vi "RunTillAbort - Luca.vi"(0 "Exposure Time (secs)":sgl, 1 "EM Advanced":i32 min=0 max=300 step=1, 2 "EM Gain":i32=1 min=1 max=300 step=1, 3 "Readout Speed (MHz)":i32 min=0 max=0, 5 "Trigger Mode":T1, 6 "Start Acquisition":bool, 8 "stop":bool, 10 "shutdown":bool) -> (4 "VS Speed (us)":sgl format="%.2f", 7 "Start Acquisition":bool, 9 "Acquiring":bool, 11 "Shut Down":bool, 19 "Intensity Graph":i32[][](graph))   [LabVIEW 2013]
uses:
  System Files/user.lib/atmcd32d.llb/TriggerMode_mode typedef.ctl
  System Files/user.lib/atmcd32d.llb/HSSpeed_type typedef.ctl
  System Files/user.lib/atmcd32d.llb/EMGainMode_mode typedef.ctl
  System Files/user.lib/atmcd32d.llb/Error Code Enum typedef.ctl
  System Files/user.lib/atmcd32d.llb/Shutter_type typedef.ctl
  System Files/user.lib/atmcd32d.llb/Shutter_mode typedef.ctl
panel:
  out "Cycle Time":sgl format="%.4f"
  out "Temperature Stable":bool
  out "Current Temperature":i32
  in  "VS Speed (us)":i32 min=0 max=0
  out "Readout Speed (MHz)":sgl format="%.2f"
  out "Start Acquisition":u32
  out "SetTriggerMode":u32
  out "SetVSSpeed":u32
  out "SetHSSpeed":u32
  out "GetMostRecentImage":u32
  out "Image Array":i32[](array[numeric]) caption="Array"
  out "Shutdown":u32
  out "GetDetector":u32
  out "Y Pixels":i32
  out "Total number of pixels":i32
  out "SetImage":u32
  out "X Pixels":i32
  out "SetExposureTime":u32
  out "SetReadMode":u32
  out "SetAcquisition Mode":u32
  out "Initialize":u32
  # "Return Values"
  # "Numerical data"
  # "INPUT"
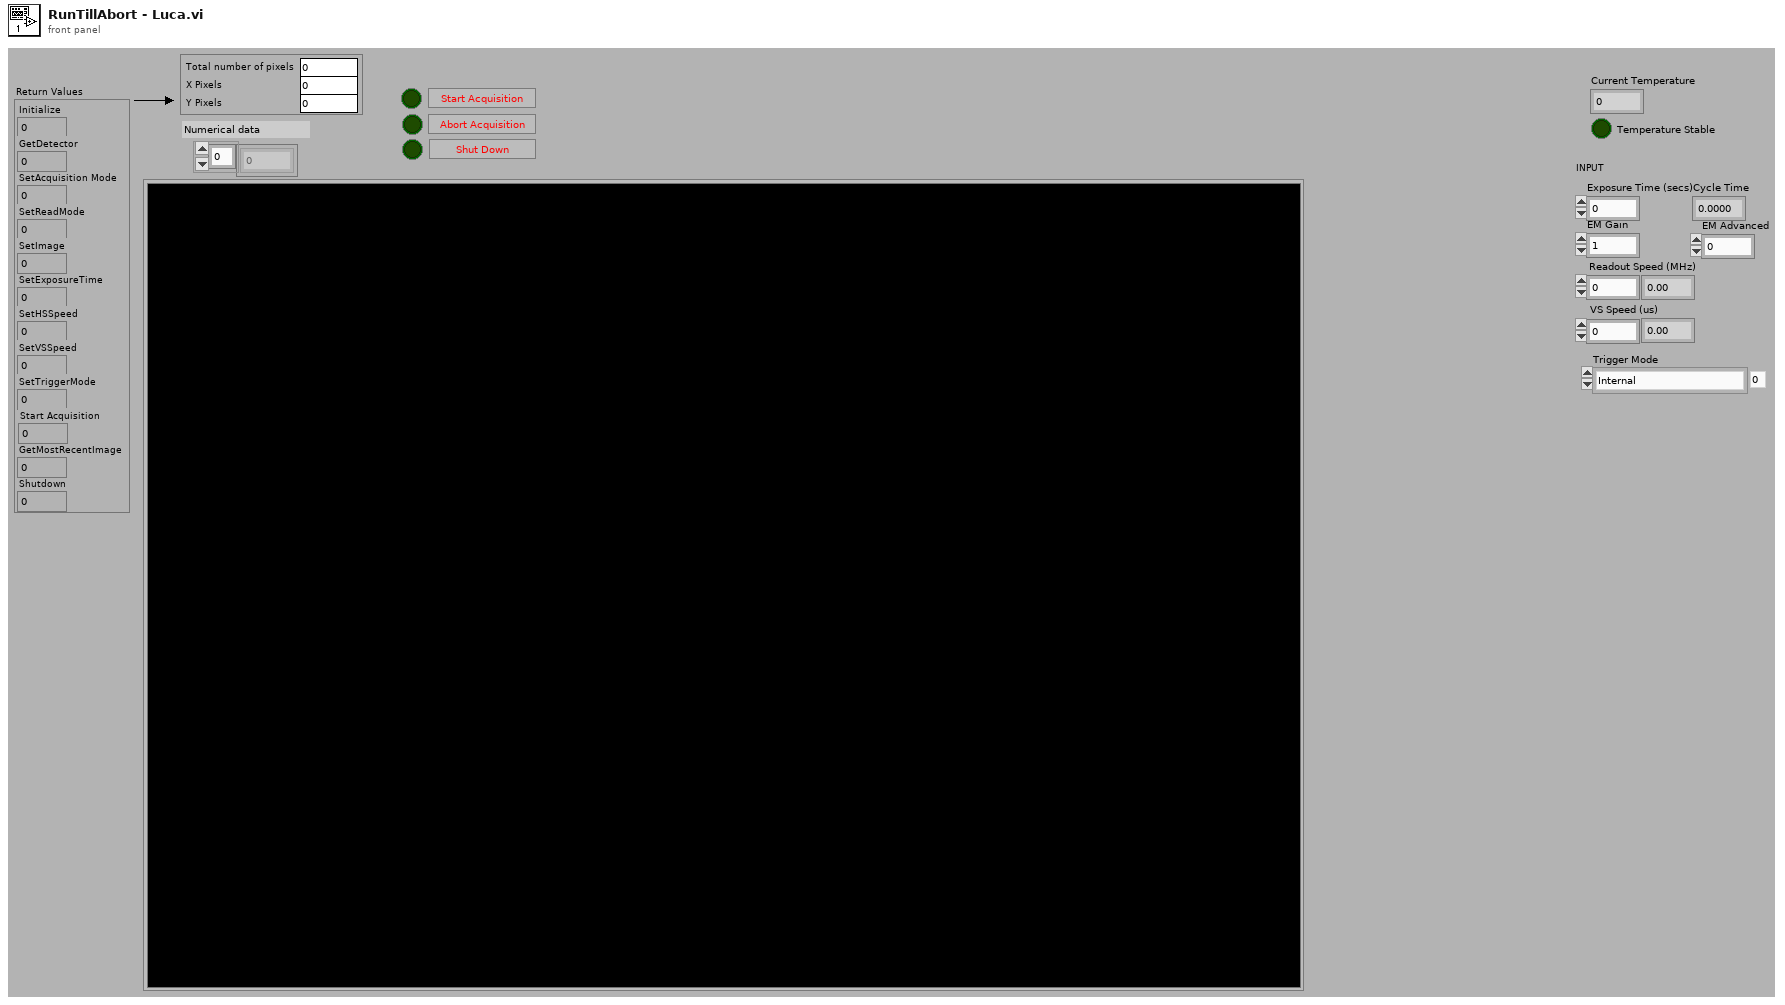
[diagram p1: front panel]
types:
  T1 = typedef "TriggerMode_mode typedef.ctl" = enum16{"Internal", "External", "N/A (2)", "N/A (3)", "N/A (4)", "N/A (5)", "External Start", "External Exposure (Bulb)", "N/A (8)", "External FVB EM", "Software", "N/A (11)", "External Charge Shifting"}
  T2 = typedef "EMGainMode_mode typedef.ctl" = enum16{"8-bit", "12-bit", "Linear", "Real"}
  T3 = typedef "Error Code Enum typedef.ctl" = enum32{"N/A (0)", "DRV_ERROR_CODES", "DRV_SUCCESS", "DRV_VXDNOTINSTALLED", "DRV_ERROR_SCAN", "DRV_ERROR_CHECK_SUM", "DRV_ERROR_FILELOAD", "DRV_UNKNOWN_FUNC", "DRV_ERROR_VXD_INIT", "DRV_ERROR_ADDRESS", "DRV_ERROR_PAGELOCK", "DRV_ERROR_PAGEUNLOCK", "DRV_ERROR_BOARDTEST", "DRV_ERROR_ACK", "DRV_ERROR_UP_FIFO", "DRV_ERROR_PATTERN", "N/A (16)", "DRV_ACQUISITION_ERRORS", "DRV_ACQ_BUFFER", "DRV_ACQ_DOWNFIFO_FULL", "DRV_PROC_UNKONWN_INSTRUCTION", "DRV_ILLEGAL_OP_CODE", "DRV_KINETIC_TIME_NOT_MET", "DRV_ACCUM_TIME_NOT_MET", "DRV_NO_NEW_DATA", "N/A (25)", "DRV_SPOOLERROR", "N/A (27)", "N/A (28)", "N/A (29)", "N/A (30)", "N/A (31)", "N/A (32)", "DRV_TEMPERATURE_CODES", "DRV_TEMPERATURE_OFF", "DRV_TEMPERATURE_NOT_STABILIZED", "DRV_TEMPERATURE_STABILIZED", "DRV_TEMPERATURE_NOT_REACHED", "DRV_TEMPERATURE_OUT_RANGE", "DRV_TEMPERATURE_NOT_SUPPORTED", "DRV_TEMPERATURE_DRIFT", "N/A (41)", "N/A (42)", "N/A (43)", "N/A (44)", "N/A (45)", "N/A (46)", "N/A (47)", "N/A (48)", "DRV_GENERAL_ERRORS", "DRV_INVALID_AUX", "DRV_COF_NOTLOADED", "DRV_FPGAPROG", "DRV_FLEXERROR", "DRV_GPIBERROR", "N/A (55)", "N/A (56)", "N/A (57)", "N/A (58)", "N/A (59)", "N/A (60)", "N/A (61)", "N/A (62)", "N/A (63)", "DRV_DATATYPE", "DRV_DRIVER_ERRORS", "DRV_P1INVALID", "DRV_P2INVALID", "DRV_P3INVALID", "DRV_P4INVALID", "DRV_INIERROR", "DRV_COFERROR", "DRV_ACQUIRING", "DRV_IDLE", "DRV_TEMPCYCLE", "DRV_NOT_INITIALIZED", "DRV_P5INVALID", "DRV_P6INVALID", "DRV_INVALID_MODE", "DRV_INVALID_FILTER", "DRV_I2CERRORS", "DRV_I2CDEVNOTFOUND", "DRV_I2CTIMEOUT", "DRV_P7INVALID", "N/A (84)", "N/A (85)", "N/A (86)", "N/A (87)", "N/A (88)", "N/A (89)", "DRV_IOCERROR", "DRV_VRMVERSIONERROR"}
  T4 = typedef "Shutter_mode typedef.ctl" = enum16{"Auto", "Open", "Close"}
  T5 = typedef "Shutter_type typedef.ctl" = enum16{"TTL Low", "TTL High"}
  T6 = typedef "HSSpeed_type typedef.ctl" = enum16{"EM Amp", "Conventional Amp"}
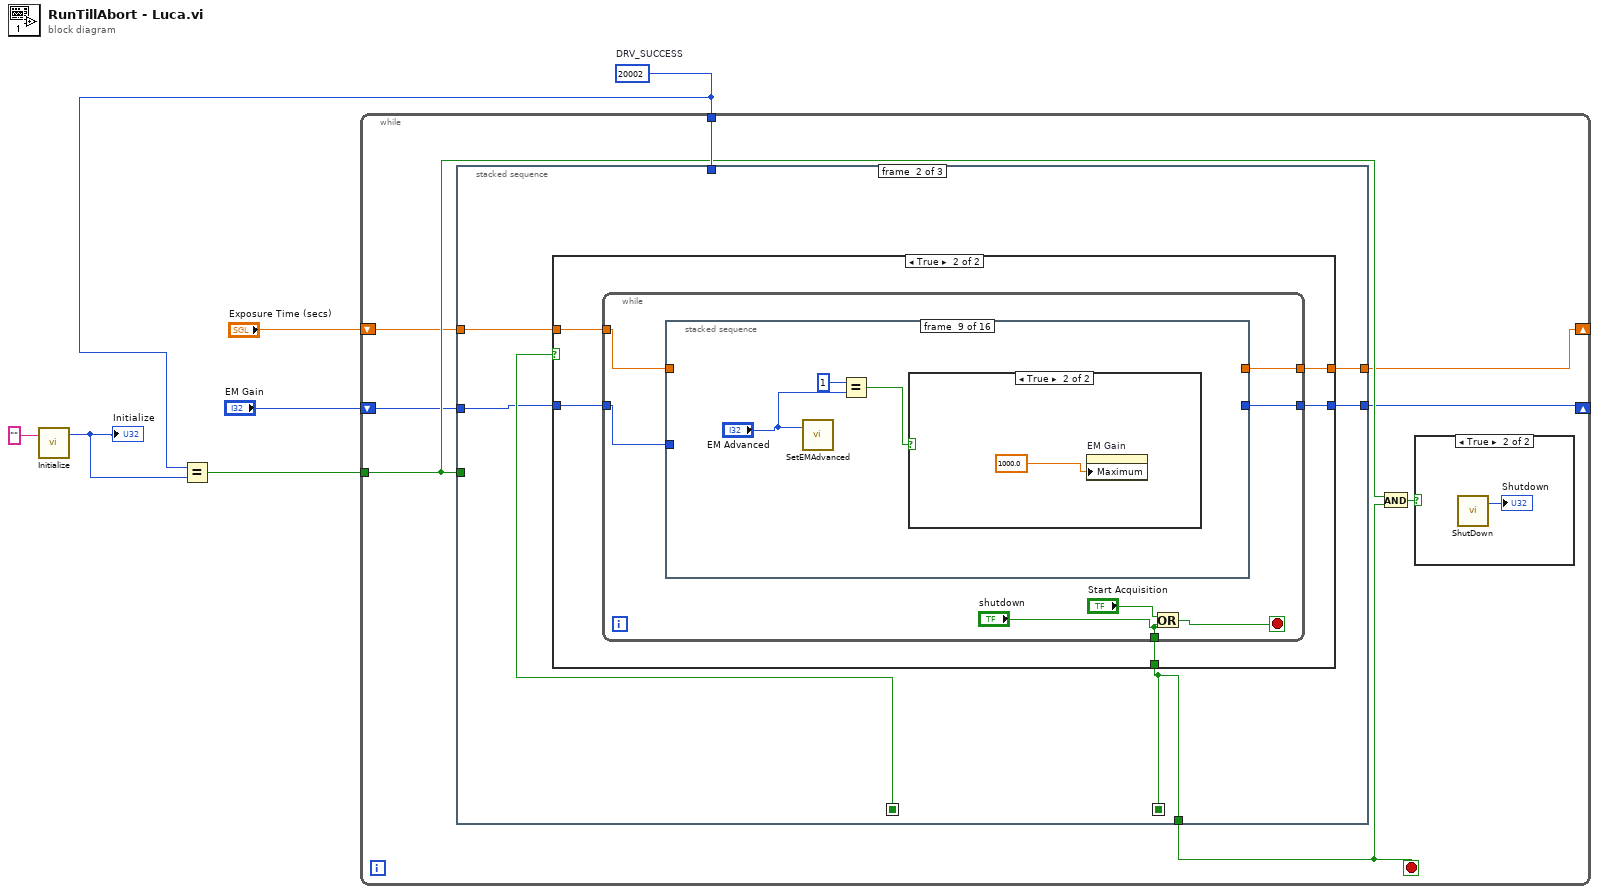
[diagram p0: block diagram]
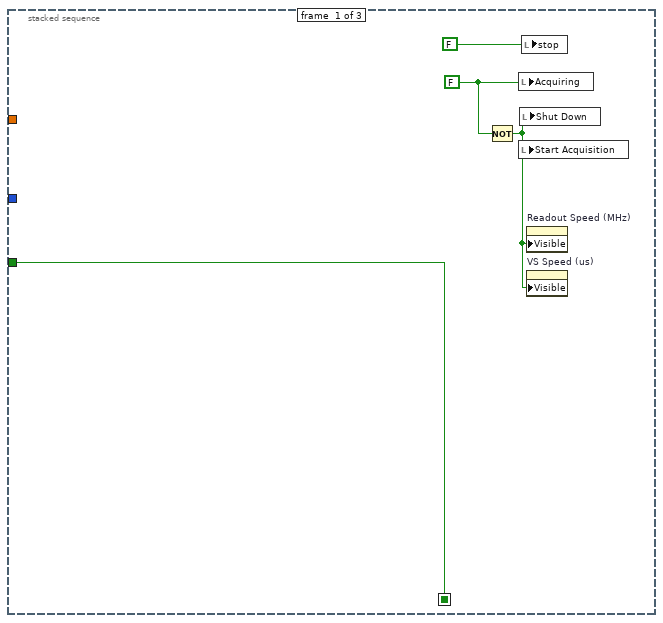
[diagram p3: hidden frame]
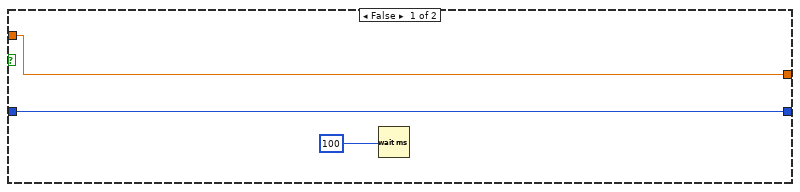
[diagram p4: hidden frame]
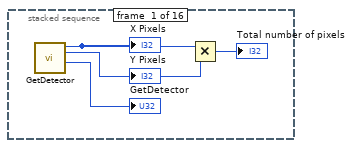
[diagram p5: hidden frame]
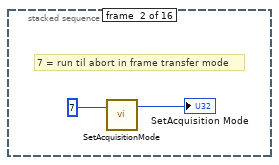
[diagram p6: hidden frame]
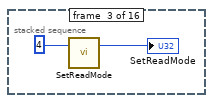
[diagram p7: hidden frame]
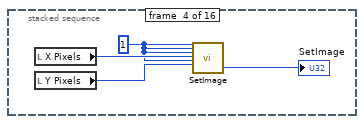
[diagram p8: hidden frame]
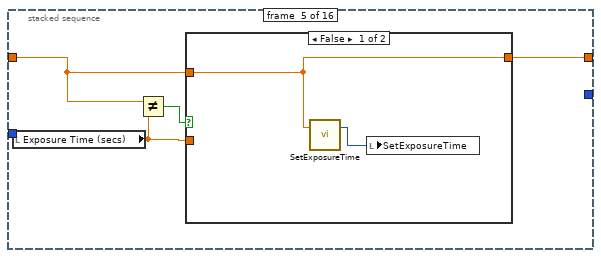
[diagram p9: hidden frame]
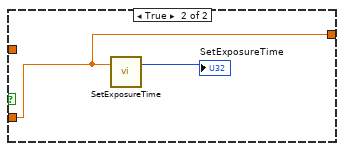
[diagram p10: hidden frame]
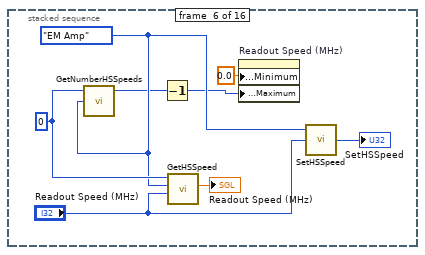
[diagram p11: hidden frame]
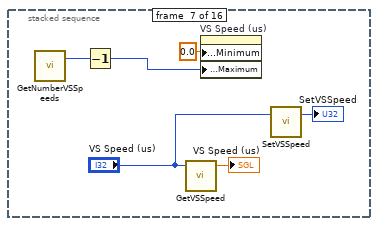
[diagram p12: hidden frame]
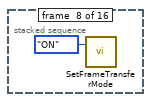
[diagram p13: hidden frame]
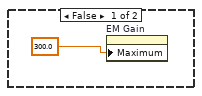
[diagram p14: hidden frame]
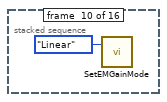
[diagram p15: hidden frame]
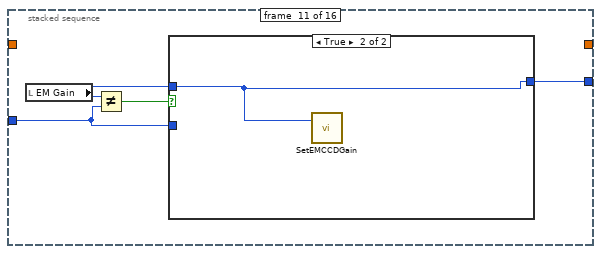
[diagram p16: hidden frame]
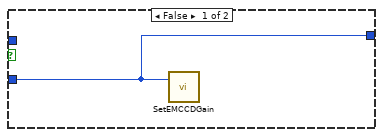
[diagram p17: hidden frame]
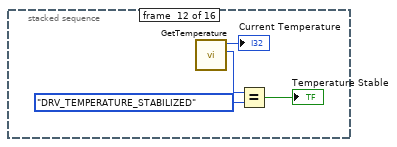
[diagram p18: hidden frame]
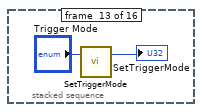
[diagram p19: hidden frame]
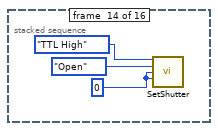
[diagram p20: hidden frame]
diagram:
  w3 = 20002  # DRV_SUCCESS
  n1 = call "Initialize.vi"("directory (\"\")"="") -> ("DLL error code"=w6:u32)  [unwired: 1 in, 1 out]
  "Initialize" <- w6
  n2 = Equal?(x=w3, y=w6) -> (x = y?=w4:bool)
  n3 = while {
    tunnel: w3 -> [w14]
    tunnel: w4 -> [w11]
    shift-right: [w8] -> _
    shift-left: "Exposure Time (secs)" -> [w10]
    shift-right: [w7] -> _
    shift-left: "EM Gain" -> [w9]
    stop <- w12 stop-if-true
    n4 = stacked-sequence {
      seq-local: [w18 _ _] -> [_ w25 w102]
      seq-local: [_ w22 _] -> [_ _ w104]
      tunnel: w14 -> [_ _ w107]
      tunnel: w9 -> [_ w24 w106]
      tunnel: w10 -> [_ w23 w105]
      tunnel: [_ w22 _] -> w12
      tunnel: w11 -> [w18 _ _]
      tunnel: [_ w21 _] -> w8
      tunnel: [_ w20 _] -> w7
      frame #0 {
        w17 = FALSE
        n5 = Not(x=w17) -> (.not. x?=w16:bool)
        n6 = local write "Acquiring"(w17) -> ()
        n7 = local write "Start Acquisition"(w16) -> ()
        n8 = local write "Shut Down"(w16) -> ()
        n9 = local write "stop"(FALSE) -> ()
        n10 = property on="Readout Speed (MHz)" class="DigNum (strict)"("Visible"=w16) -> ()  [unwired: 2 in, 2 out]
        n11 = property on="VS Speed (us)" class="DigNum (strict)"("Visible"=w16) -> ()  [unwired: 2 in, 2 out]
      }
      frame #1 {
        n12 = case shown="True" w25 {
          tunnel: w24 -> [w26 w33]
          tunnel: w23 -> [w27 w32]
          tunnel: [_ w31] -> w22
          tunnel: [w27 w30] -> w21
          tunnel: [w26 w29] -> w20
          frame False {
            n13 = Wait (ms)(milliseconds to wait=100) -> ()  [unwired: 1 out]
          }
          frame True {
            n14 = while {
              tunnel: w33 -> [w40]
              tunnel: w32 -> [w39]
              tunnel: ["shutdown"] -> w31
              tunnel: [w35] -> w30
              tunnel: [w34] -> w29
              stop <- w37 stop-if-true
              n15 = stacked-sequence {
                tunnel: w40 -> [_ _ _ _ _ _ _ _ _ _ w83 _ _ _ _ _]
                tunnel: w39 -> [_ _ _ _ w53 _ _ _ _ _ _ _ _ _ _ _]
                tunnel: [_ _ _ _ w54 _ _ _ _ _ _ _ _ _ _ _] -> w35
                tunnel: [_ _ _ _ _ _ _ _ _ _ w82 _ _ _ _ _] -> w34
                frame #0 {
                  n16 = call "GetDetector.vi"() -> ("DLL error code"=→"GetDetector":u32, "ypixels"=w43:i32, "xpixels"=w42:i32)  [unwired: 4 in, 1 out]
                  "X Pixels" <- w42
                  "Y Pixels" <- w43
                  n17 = Multiply(x=w42, y=w43) -> (x*y=→"Total number of pixels":i32)
                }
                frame #1 {
                  # "7 = run til abort in frame transfer mode"
                  n18 = call "SetAcquisitionMode.vi"("mode"=u16 7 ("AcquisitionMode")) -> ("DLL error code"=→"SetAcquisition Mode":u32)  [unwired: 1 in, 1 out]
                }
                frame #2 {
                  n19 = call "SetReadMode.vi"("mode"=u16 4 ("ReadMode")) -> ("DLL error code"=→"SetReadMode":u32)  [unwired: 1 in, 1 out]
                }
                frame #3 {
                  w51 = 1
                  n20 = local read "X Pixels"() -> (w52:i32)
                  n21 = local read "Y Pixels"() -> (w50:i32)
                  n22 = call "SetImage.vi"("hbin"=w51, "vbin"=w51, "hstart"=w51, "hend"=w52, "vstart"=w51, "vend"=w50) -> ("DLL error code"=→"SetImage":u32)  [unwired: 20 in, 1 out]
                }
                frame #4 {
                  n23 = local read "Exposure Time (secs)"() -> (w55:sgl)
                  n24 = Not Equal?(x=w53, y=w55) -> (x != y?=w56:bool)
                  n25 = case shown="False" w56 {
                    tunnel: w55 -> [_ w59]
                    tunnel: [w57 w59] -> w54
                    tunnel: w53 -> [w57 _]
                    frame False {
                      n26 = call "SetExposureTime.vi"("time"=w57) -> ("DLL error code"=w58:u32)  [unwired: 1 in, 1 out]
                      n27 = local write "SetExposureTime"(w58) -> ()
                    }
                    frame True {
                      n28 = call "SetExposureTime.vi"("time"=w59) -> ("DLL error code"=→"SetExposureTime":u32)  [unwired: 1 in, 1 out]
                    }
                  }
                }
                frame #5 {
                  w67 = 0 ("channel")
                  w66 = HSSpeed_type_typedef."EM Amp" ("type")
                  n29 = call "GetNumberHSSpeeds.vi"("type"=w66, "channel"=w67) -> ("number"=w64:i32)  [unwired: 1 in, 2 out]
                  n30 = Decrement(x=w64) -> (x-1=w63:i32)
                  n31 = call "GetHSSpeed.vi"("index"="Readout Speed (MHz)", "type"=w66, "channel"=w67) -> ("speed"=→"Readout Speed (MHz)":sgl)  [unwired: 2 in, 2 out]
                  n32 = property on="Readout Speed (MHz)" class="DigNum (strict)"("Data Range:Minimum"=0.0, "Data Range:Maximum"=w63) -> ()  [unwired: 2 in, 2 out]
                  n33 = call "SetHSSpeed.vi"("index"="Readout Speed (MHz)", "type"=w66) -> ("DLL error code"=→"SetHSSpeed":u32)  [unwired: 2 in, 1 out]
                }
                frame #6 {
                  n34 = call "GetNumberVSSpeeds.vi"() -> ("number"=w69:i32)  [unwired: 3 in, 2 out]
                  n35 = Decrement(x=w69) -> (x-1=w70:i32)
                  n36 = call "GetVSSpeed.vi"("index"="VS Speed (us)") -> ("speed"=→"VS Speed (us)":sgl)  [unwired: 2 in, 2 out]
                  n37 = property on="VS Speed (us)" class="DigNum (strict)"("Data Range:Minimum"=0.0, "Data Range:Maximum"=w70) -> ()  [unwired: 2 in, 2 out]
                  n38 = call "SetVSSpeed.vi"("index"="VS Speed (us)") -> ("DLL error code"=→"SetVSSpeed":u32)  [unwired: 1 in, 1 out]
                }
                frame #7 {
                  n39 = call "SetFrameTransferMode.vi"("mode"=enum16{"OFF", "ON"}."ON") -> ()  [unwired: 1 in, 2 out]
                }
                frame #8 {
                  n40 = call "SetEMAdvanced.vi"("state"="EM Advanced") -> ()  [unwired: 1 in, 2 out]
                  n41 = Equal?(x=1, y="EM Advanced") -> (x = y?=w78:bool)
                  n42 = case shown="True" w78 {
                    frame False {
                      n43 = property on="EM Gain" class="DigNum (strict)"("Maximum"=300.0 ("Data Range:Maximum")) -> ()  [unwired: 2 in, 2 out]
                    }
                    frame True {
                      n44 = property on="EM Gain" class="DigNum (strict)"("Maximum"=1000.0 ("Data Range:Maximum")) -> ()  [unwired: 2 in, 2 out]
                    }
                  }
                }
                frame #9 {
                  n45 = call "SetEMGainMode.vi"("mode"=EMGainMode_mode_typedef."Linear") -> ()  [unwired: 1 in, 2 out]
                }
                frame #10 {
                  n46 = local read "EM Gain"() -> (w84:i32)
                  n47 = Not Equal?(x=w84, y=w83) -> (x != y?=w85:bool)
                  n48 = case shown="True" w85 {
                    tunnel: w84 -> [_ w87]
                    tunnel: w83 -> [w86 _]
                    tunnel: [w86 w87] -> w82
                    frame False {
                      n49 = call "SetEMCCDGain.vi"("gain"=w86) -> ()  [unwired: 1 in, 2 out]
                    }
                    frame True {
                      n50 = call "SetEMCCDGain.vi"("gain"=w87) -> ()  [unwired: 1 in, 2 out]
                    }
                  }
                }
                frame #11 {
                  n51 = call "GetTemperature.vi"() -> ("status"=w90:T3, "temperature"=→"Current Temperature":i32)  [unwired: 4 in, 2 out]
                  n52 = Equal?(x=w90, y=Error_Code_Enum_typedef."DRV_TEMPERATURE_STABILIZED") -> (x = y?=→"Temperature Stable":bool)
                }
                frame #12 {
                  n53 = call "SetTriggerMode.vi"("mode"="Trigger Mode") -> ("DLL error code"=→"SetTriggerMode":u32)  [unwired: 1 in, 1 out]
                }
                frame #13 {
                  w94 = 0 ("closingtime (0)")
                  n54 = call "SetShutter.vi"("type"=Shutter_type_typedef."TTL High", "mode"=Shutter_mode_typedef."Open", "closingtime"=w94, "openingtime"=w94) -> ()  [unwired: 10 in, 2 out]
                }
                frame #14 {
                  n55 = local read "Total number of pixels"() -> (w98:i32)
                  n56 = Initialize Array(0, w98) -> (w97:i32[])
                  n57 = local write "Image Array"(w97) -> ()
                }
                frame #15 {
                  n58 = call "GetAcquisitionTimings.vi"() -> ("exposure"=→"Cycle Time":sgl)  [unwired: 11 in, 4 out]
                }
              }
              n59 = Or(x="Start Acquisition", y="shutdown") -> (x .or. y?=w37:bool)
            }
          }
        }
      }
      frame #2 {
        n60 = Not(x=w104) -> (.not. x?=w103:bool)
        n61 = And(x=w102, y=w103) -> (x .and. y?=w101:bool)
        n62 = case shown="True" w101 {
          tunnel: w107 -> [_ w111]
          tunnel: w106 -> [_ w110]
          tunnel: w105 -> [_ w109]
          frame False {
            n63 = Wait (ms)(milliseconds to wait=100) -> ()  [unwired: 1 out]
          }
          frame True {
            n64 = stacked-sequence {
              tunnel: w111 -> [_ w117 _]
              tunnel: w110 -> [_ w116 _]
              tunnel: w109 -> [_ w115 _]
              frame #0 {
                n65 = call "StartAcquisition.vi"() -> ("DLL error code"=w112:u32)  [unwired: 2 in, 1 out]
                n66 = local write "Start Acquisition"(w112) -> ()
              }
              frame #1 {
                w114 = TRUE
                n67 = while {
                  tunnel: w117 -> [w122]
                  shift-right: [w121] -> _
                  shift-left: w116 -> [w118]
                  shift-right: [w120] -> _
                  shift-left: w115 -> [w119]
                  stop <- w123 stop-if-true
                  n68 = stacked-sequence {
                    tunnel: ["stop" _] -> w123
                    tunnel: w122 -> [w124 _]
                    tunnel: [_ w144] -> w121
                    tunnel: w119 -> [_ w141]
                    tunnel: [_ w142] -> w120
                    tunnel: w118 -> [_ w143]
                    frame #0 {
                      n69 = while {
                        tunnel: [w135] -> w130
                        tunnel: w124 -> [w132]
                        stop <- w138 stop-if-true
                        n70 = local read "Total number of pixels"() -> (w137:i32)
                        n71 = local read "Image Array"() -> (w136:i32[])
                        n72 = call "GetMostRecentImage.vi"("size"=w137, "array"=w136) -> ("array"=w135:i32[], "DLL error code"=w133:u32)  [unwired: 1 in, 1 out]
                        "GetMostRecentImage" <- w133
                        n73 = local read "stop"() -> (w134:bool)
                        n74 = Equal?(x=w132, y=w133) -> (x = y?=w131:bool)
                        n75 = Or(x=w134, y=w131) -> (x .or. y?=w138:bool)
                        n76 = Wait (ms)(milliseconds to wait=25) -> ()  [unwired: 1 out]
                      }
                      "Image Array" <- w130
                      n77 = Not(x="stop") -> (.not. x?=w126:bool)
                      n78 = local write "Acquiring"(w126) -> ()
                      n79 = local read "Y Pixels"() -> (w128:i32)
                      n80 = local read "X Pixels"() -> (w127:i32)
                      n81 = Reshape Array(w130, w128, w127) -> (→"Intensity Graph":i32[][])
                    }
                    frame #1 {
                      n82 = local read "Exposure Time (secs)"() -> (w140:sgl)
                      n83 = local read "EM Gain"() -> (w145:i32)
                      n84 = Not Equal?(x=w145, y=w143) -> (x != y?=w147:bool)
                      n85 = Not Equal?(x=w141, y=w140) -> (x != y?=w148:bool)
                      n86 = Or(x=w148, y=w147) -> (x .or. y?=w146:bool)
                      n87 = case shown="True" w146 {
                        tunnel: w145 -> [_ w154]
                        tunnel: [w150 w153] -> w144
                        tunnel: w143 -> [w150 _]
                        tunnel: w140 -> [_ w152]
                        tunnel: [w149 w151] -> w142
                        tunnel: w141 -> [w149 _]
                        frame False {
                        }
                        frame True {
                          n88 = stacked-sequence {
                            tunnel: w154 -> [_ w155 _ _ _]
                            tunnel: [_ w155 _ _ _] -> w153
                            tunnel: w152 -> [_ _ w156 _ _]
                            tunnel: [_ _ w156 _ _] -> w151
                            frame #0 {
                              n89 = call "AbortAcquisition.vi"() -> ()  [unwired: 2 in, 2 out]
                            }
                            frame #1 {
                              n90 = call "SetEMCCDGain.vi"("gain"=w155) -> ()  [unwired: 1 in, 2 out]
                            }
                            frame #2 {
                              n91 = call "SetExposureTime.vi"("time"=w156) -> ()  [unwired: 1 in, 2 out]
                            }
                            frame #3 {
                              n92 = call "GetAcquisitionTimings.vi"() -> ("exposure"=w157:sgl)  [unwired: 11 in, 4 out]
                              n93 = local write "Cycle Time"(w157) -> ()
                            }
                            frame #4 {
                              n94 = call "StartAcquisition.vi"() -> ("DLL error code"=→"Start Acquisition":u32)  [unwired: 2 in, 1 out]
                            }
                          }
                        }
                      }
                    }
                  }
                }
                n95 = Not(x=w114) -> (.not. x?=w113:bool)
                "Start Acquisition" <- w113
                "Shut Down" <- w113
                n96 = property on="Readout Speed (MHz)" class="DigNum (strict)"("Visible"=w113) -> ()  [unwired: 2 in, 2 out]
                n97 = property on="VS Speed (us)" class="DigNum (strict)"("Visible"=w113) -> ()  [unwired: 2 in, 2 out]
                "Acquiring" <- w114
              }
              frame #2 {
                n98 = call "AbortAcquisition.vi"() -> ()  [unwired: 2 in, 2 out]
              }
            }
          }
        }
      }
    }
    n99 = And(x=w11, y=w12) -> (x .and. y?=w13:bool)
    n100 = case shown="True" w13 {
      frame False {
      }
      frame True {
        n101 = call "ShutDown.vi"() -> ("DLL error code"=→"Shutdown":u32)  [unwired: 2 in, 1 out]
      }
    }
  }
